vi "Test draw root.vi"() -> ()   [LabVIEW 2020]
panel:
  in  "Point 3":refnum<k7>
  in  "Point 2":refnum<k7>
  in  "LinePattern":refnum<k7>
  out "layer_handle":i32
  in  "CurrentZoom":i32
  in  "Lon":dbl
  in  "Lat":dbl
  out "ProjY":dbl format="%.2f"
  out "ProjX":dbl format="%#.2f"
  in  "CursorMode 2":i32(ring) items=["cmZoomIn"=0, "cmZoomOut"=1, "cmPan"=2, "cmSelection"=3, "cmNone"=4, "cmMeasure"=5, "cmAddShape"=6, "cmEditShape"=8, "cmSplitByPolyline"=9, "cmIdentify"=10, "cmMoveShapes"=11, "cmRotateShapes"=12, "cmSelectByPolygon"=13, "cmEraseByPolygon"=14, "cmSplitByPolygon"=15, "cmClipByPolygon"=16]
  out "degreesLatY":dbl
  out "degreesLngX":dbl
  in  "stop":bool
  in  "Point":refnum<k7>
  in  "Shape":refnum<k7>
  in  "Shapefile":refnum<k7>
  in  "Map":refnum<k7>(container)
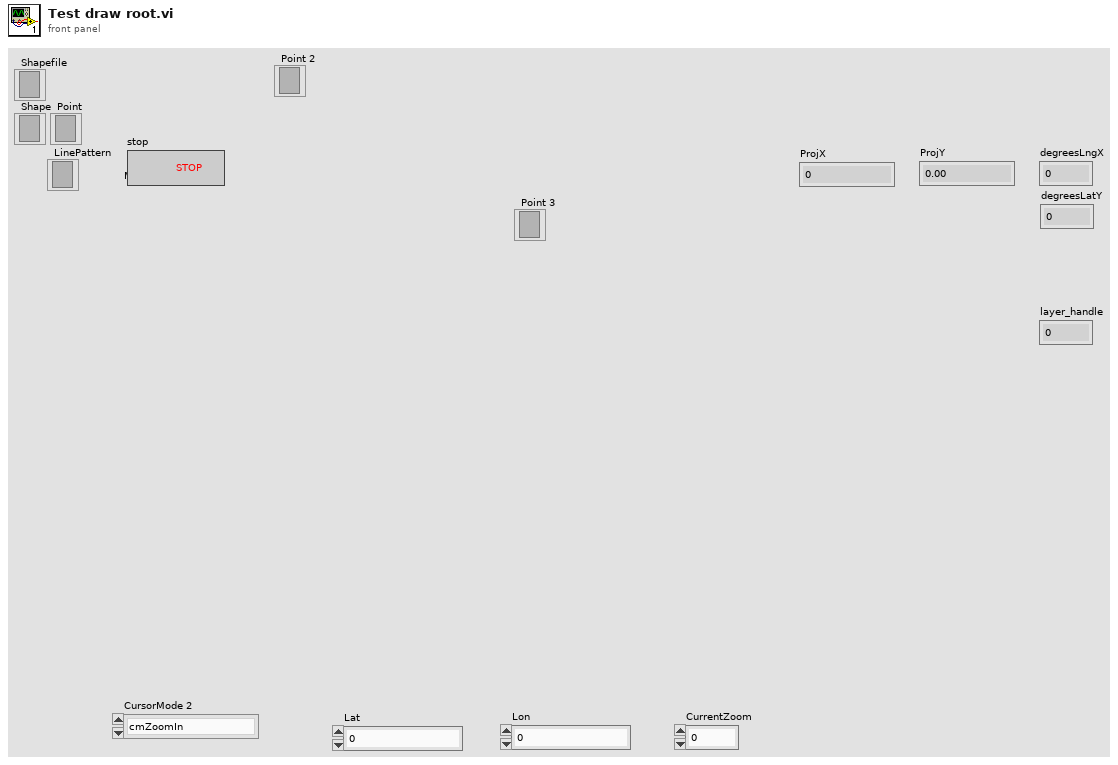
[diagram p1: front panel]
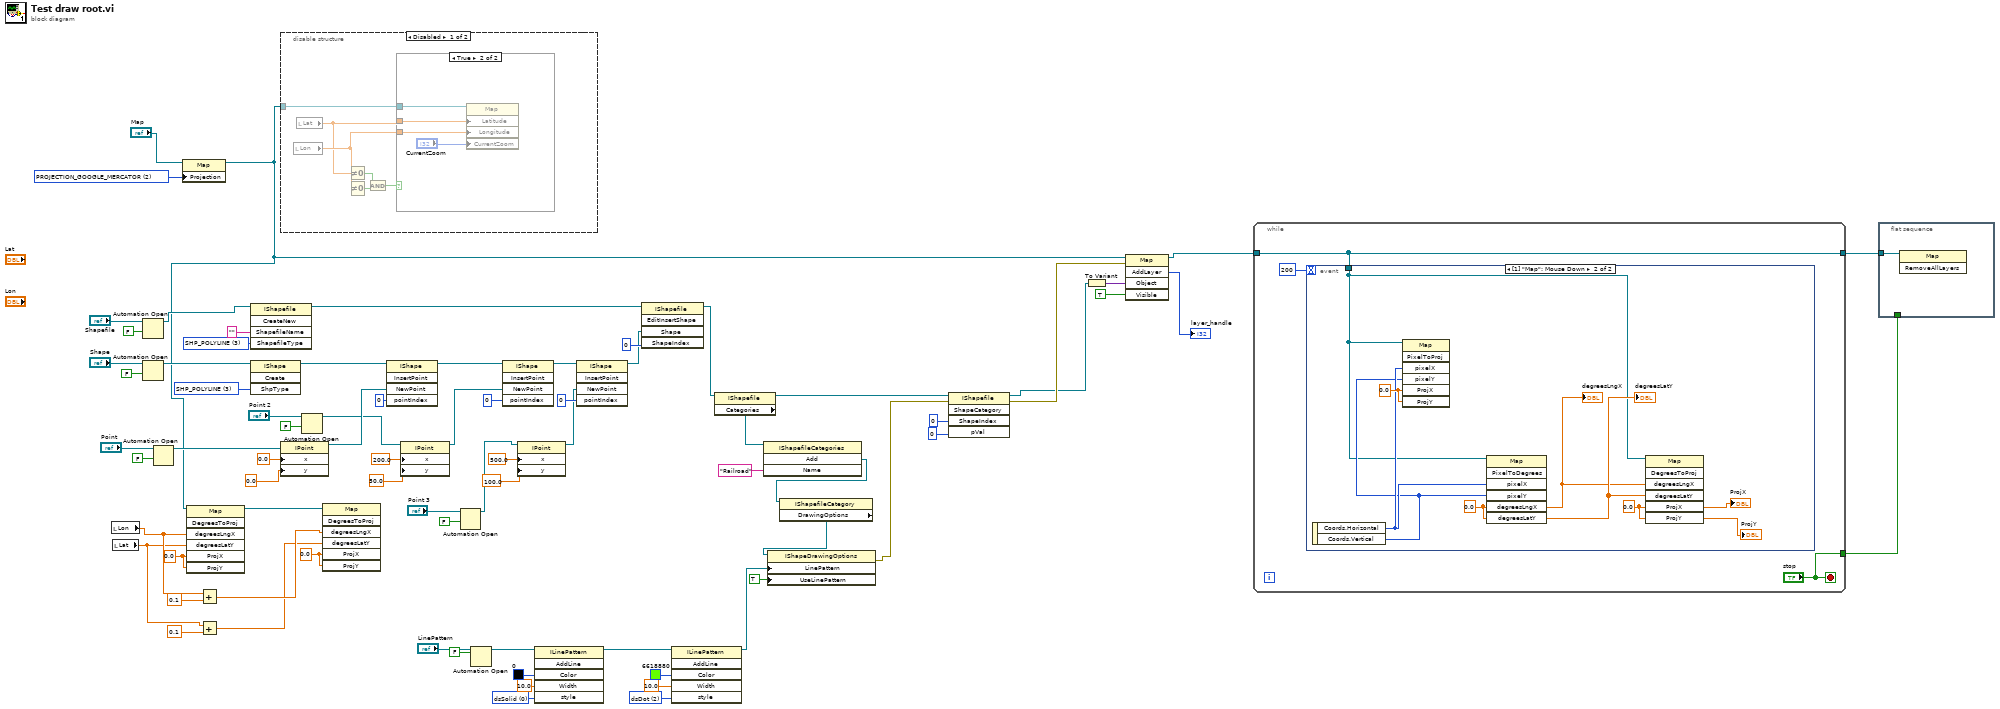
[diagram p0: block diagram]
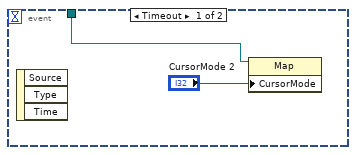
[diagram p4: hidden frame]
diagram:
  w28 = 2 items=["dsSolid", "dsDash", "dsDot", "dsDashDot", "dsDashDotDot", "dsCustom"] ("style")
  w32 = 0 items=["dsSolid", "dsDash", "dsDot", "dsDashDot", "dsDashDotDot", "dsCustom"] ("style")
  w56 = 0.0 ("ProjX")
  w63 = 0.0 ("ProjX")
  w64 = 2 items=["PROJECTION_CUSTOM"=-1, "PROJECTION_NONE"=0, "PROJECTION_WGS84"=1, "PROJECTION_GOOGLE_MERCATOR"=2] ("Projection")
  w67 = 3 items=["SHP_NULLSHAPE"=0, "SHP_POINT"=1, "SHP_POLYLINE"=3, "SHP_POLYGON"=5, "SHP_MULTIPOINT"=8, "SHP_POINTZ"=11, "SHP_POLYLINEZ"=13, "SHP_POLYGONZ"=15, "SHP_MULTIPOINTZ"=18, "SHP_POINTM"=21, "SHP_POLYLINEM"=23, "SHP_POLYGONM"=25, "SHP_MULTIPOINTM"=28, "SHP_MULTIPATCH"=31] ("ShpType")
  w69 = 3 items=["SHP_NULLSHAPE"=0, "SHP_POINT"=1, "SHP_POLYLINE"=3, "SHP_POLYGON"=5, "SHP_MULTIPOINT"=8, "SHP_POINTZ"=11, "SHP_POLYLINEZ"=13, "SHP_POLYGONZ"=15, "SHP_MULTIPOINTZ"=18, "SHP_POINTM"=21, "SHP_POLYLINEM"=23, "SHP_POLYGONM"=25, "SHP_MULTIPOINTM"=28, "SHP_MULTIPATCH"=31] ("ShapefileType")
  n1 = local read "Lon"() -> (w55:dbl)
  n2 = local read "Lat"() -> (w51:dbl)
  n3 = Automation Open(Automation Refnum="Shapefile", 9:FALSE ("open new instance (false)")) -> (Automation Refnum=w71:refnum<k7>)  [unwired: 2 in, 1 out]
  n4 = Automation Open(Automation Refnum="Shape", 9:FALSE ("open new instance (false)")) -> (Automation Refnum=w68:refnum<k7>)  [unwired: 2 in, 1 out]
  n5 = Automation Open(Automation Refnum="Point", 9:FALSE ("open new instance (false)")) -> (Automation Refnum=w66:refnum<k7>)  [unwired: 2 in, 1 out]
  n6 = property class="Map"(reference="Map", "Projection"=w64) -> (reference out=w43:refnum<k7>)  [unwired: 1 in, 1 out]
  n7 = invoke class="Map" method="DegreesToProj"(reference=w43, "degreesLngX"=w55, "degreesLatY"=w51, "ProjX"=w63, "ProjY"=w63) -> (reference out=w60:refnum<k7>)  [unwired: 2 in, 6 out]
  n8 = Add(x=w55, y=0.1) -> (x+y=w53:dbl)
  n9 = Add(x=w51, y=0.1) -> (x+y=w50:dbl)
  n10 = invoke class="IShapefile" method="CreateNew"(reference=w71, "ShapefileName"="", "ShapefileType"=w69) -> (reference out=w49:refnum<k7>)  [unwired: 2 in, 4 out]
  n11 = invoke class="IShape" method="Create"(reference=w68, "ShpType"=w67) -> (reference out=w61:refnum<k7>)  [unwired: 2 in, 3 out]
  n12 = disable-structure shown="Disabled" {
    disable-tunnel: w43 -> [w78 _]
    frame Disabled {
      n13 = local read "Lon"() -> (w83:dbl)
      n14 = local read "Lat"() -> (w82:dbl)
      n15 = Not Equal To 0?(x=w82) -> (x != 0?=w79:bool)
      n16 = Not Equal To 0?(x=w83) -> (x != 0?=w80:bool)
      n17 = And(x=w79, y=w80) -> (x .and. y?=w81:bool)
      n18 = case shown="True" w81 {
        tunnel: w82 -> [_ w87]
        tunnel: w83 -> [_ w86]
        tunnel: w78 -> [_ w84]
        frame False {
        }
        frame True {
          n19 = property class="Map"(reference=w84, "Latitude"=w87, "Longitude"=w86, "CurrentZoom"="CurrentZoom") -> ()  [unwired: 1 in, 2 out]
        }
      }
    }
    frame Enabled {
    }
  }
  n20 = property class="IPoint"(reference=w66, "x"=0.0, "y"=0.0) -> (reference out=w12:refnum<k7>)  [unwired: 1 in, 1 out]
  n21 = Automation Open(Automation Refnum="Point 2", 9:FALSE ("open new instance (false)")) -> (Automation Refnum=w11:refnum<k7>)  [unwired: 2 in, 1 out]
  n22 = invoke class="Map" method="DegreesToProj"(reference=w60, "degreesLngX"=w53, "degreesLatY"=w50, "ProjX"=w56, "ProjY"=w56) -> ()  [unwired: 2 in, 7 out]
  n23 = invoke class="IShape" method="InsertPoint"(reference=w61, "NewPoint"=w12, "pointIndex"=0) -> (reference out=w58:refnum<k7>)  [unwired: 2 in, 4 out]
  n24 = property class="IPoint"(reference=w11, "x"=200.0, "y"=50.0) -> (reference out=w59:refnum<k7>)  [unwired: 1 in, 1 out]
  n25 = Automation Open(Automation Refnum="Point 3", 9:FALSE ("open new instance (false)")) -> (Automation Refnum=w6:refnum<k7>)  [unwired: 2 in, 1 out]
  n26 = Automation Open(Automation Refnum="LinePattern", 9:FALSE ("open new instance (false)")) -> (Automation Refnum=w35:refnum<k7>)  [unwired: 2 in, 1 out]
  n27 = invoke class="IShape" method="InsertPoint"(reference=w58, "NewPoint"=w59, "pointIndex"=0) -> (reference out=w5:refnum<k7>)  [unwired: 2 in, 4 out]
  n28 = property class="IPoint"(reference=w6, "x"=500.0, "y"=100.0) -> (reference out=w3:refnum<k7>)  [unwired: 1 in, 1 out]
  n29 = invoke class="ILinePattern" method="AddLine"(reference=w35, "Color"=u32 0, "Width"=sgl 10.0, "style"=w32) -> (reference out=w31:refnum<k7>)  [unwired: 2 in, 5 out]
  n30 = invoke class="IShape" method="InsertPoint"(reference=w5, "NewPoint"=w3, "pointIndex"=0) -> (reference out=w2:refnum<k7>)  [unwired: 2 in, 4 out]
  n31 = invoke class="IShapefile" method="EditInsertShape"(reference=w49, "Shape"=w2, "ShapeIndex"=0) -> (reference out=w42:refnum<k7>)  [unwired: 2 in, 4 out]
  n32 = invoke class="ILinePattern" method="AddLine"(reference=w31, "Color"=u32 6618880, "Width"=sgl 10.0, "style"=w28) -> (reference out=w27:refnum<k7>)  [unwired: 2 in, 5 out]
  n33 = property class="IShapefile"(reference=w42) -> (reference out=w25:refnum<k7>, "Categories"=w41:refnum<k7>)  [unwired: 1 in, 1 out]
  n34 = invoke class="IShapefileCategories" method="Add"(reference=w41, "Name"="Railroad") -> ("Add"=w39:refnum<k7>)  [unwired: 2 in, 3 out]
  n35 = property class="IShapefileCategory"(reference=w39) -> ("DrawingOptions"=w38:refnum<k7>)  [unwired: 1 in, 2 out]
  n36 = property class="IShapeDrawingOptions"(reference=w38, "LinePattern"=w27, "UseLinePattern"=TRUE) -> (error out=w24:errorcluster)  [unwired: 1 in, 1 out]
  n37 = invoke class="IShapefile" method="ShapeCategory"(reference=w25, error in=w24, "ShapeIndex"=0, "pVal"=0) -> (reference out=w1:refnum<k7>, error out=w21:errorcluster)  [unwired: 1 in, 3 out]
  n38 = To Variant(anything=w1) -> (Variant=w47:variant)
  n39 = invoke class="Map" method="AddLayer"(reference=w43, error in=w21, "Object"=w47, "Visible"=TRUE) -> (reference out=w44:refnum<k7>, "AddLayer"=→"layer_handle":i32)  [unwired: 1 in, 3 out]
  n40 = while {
    tunnel: w44 -> [w89]
    tunnel: [w89] -> w14
    tunnel: ["stop"] -> w13
    stop <- "stop" stop-if-true
    n41 = event shown="[1] \"Map\": Mouse Down" {
      selector: _ -> [_ _]
      dyn-events: _ -> [_ _]
      timeout: 200 -> [_ _]
      tunnel: w89 -> [w92 w93]
      event Timeout {
        n42 = event-data() -> ()  [unwired: 1 in, 3 out]
        n43 = property class="Map"(reference=w92, "CursorMode"="CursorMode 2") -> ()  [unwired: 1 in, 2 out]
      }
      event "Map": Mouse Down {
        w96 = 0.0 ("ProjX")
        w101 = 0.0 ("ProjX")
        w102 = 0.0 ("degreesLngX")
        n44 = event-data() -> ("Coords.Horizontal"=w100:i32, "Coords.Vertical"=w99:i32)  [unwired: 1 in]
        n45 = invoke class="Map" method="PixelToProj"(reference=w93, "pixelX"=w100, "pixelY"=w99, "ProjX"=w101, "ProjY"=w101) -> ()  [unwired: 2 in, 7 out]
        n46 = invoke class="Map" method="PixelToDegrees"(reference=w93, "pixelX"=w100, "pixelY"=w99, "degreesLngX"=w102, "degreesLatY"=w102) -> ("degreesLngX"=w97:dbl, "degreesLatY"=w98:dbl)  [unwired: 2 in, 5 out]
        "degreesLngX" <- w97
        "degreesLatY" <- w98
        n47 = invoke class="Map" method="DegreesToProj"(reference=w93, "degreesLngX"=w97, "degreesLatY"=w98, "ProjX"=w96, "ProjY"=w96) -> ("ProjX"=→"ProjX":dbl, "ProjY"=→"ProjY":dbl)  [unwired: 2 in, 5 out]
      }
    }
  }
  n48 = flat-sequence {
    tunnel: w14 -> [w103]
    tunnel: w13 -> [_]
    frame #0 {
      n49 = invoke class="Map" method="RemoveAllLayers"(reference=w103) -> ()  [unwired: 2 in, 3 out]
    }
  }
